vi "Sort Transposed Time Series Data.vi"(4 "Arrays in":dbl[][](array[numeric])) -> (1 "Arrays out":dbl[][](array[numeric]))   [LabVIEW 2013, in "Data Log Fetcher.lvlib"]
uses:
  Data Log Fetcher.lvlib
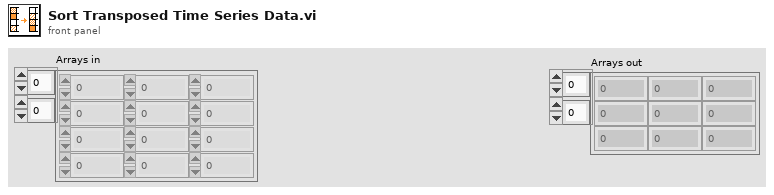
[diagram p1: front panel]
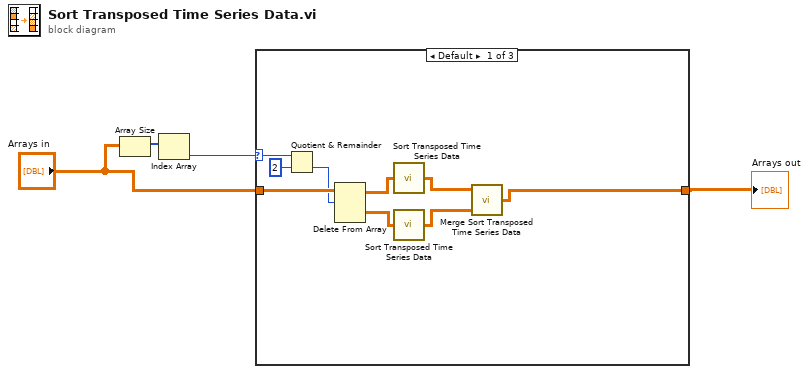
[diagram p0: block diagram]
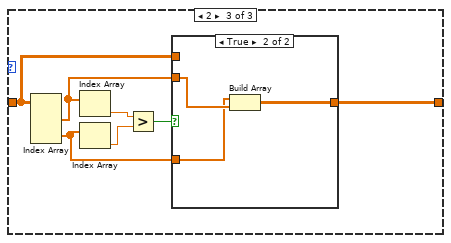
[diagram p3: hidden frame]
diagram:
  n1 = Array Size(array="Arrays in") -> (size(s)=w4:i32[])
  n2 = Index Array(array=w4) -> (element=w3:i32)  [unwired: 1 in]
  n3 = case shown="Default" w3 {
    selector: w3 -> [w12 _ _]
    tunnel: "Arrays in" -> [w13 w14 w15]
    tunnel: [w10 w14 w21] -> w2
    frame Default {
      n4 = Quotient & Remainder(x=w12, y=2) -> (floor(x/y)=w9:i32)  [unwired: 1 out]
      n5 = Delete From Array(array=w13, length=w9) -> (deleted portion=w7:dbl[][], array with subset deleted=w8:dbl[][])  [unwired: 2 in]
      n6 = call "Sort Transposed Time Series Data.vi"("Arrays in"=w8) -> ("Arrays out"=w6:dbl[][])  [unwired: 4 in]
      n7 = call "Sort Transposed Time Series Data.vi"("Arrays in"=w7) -> ("Arrays out"=w5:dbl[][])  [unwired: 4 in]
      n8 = call "Merge Sort Transposed Time Series Data.vi"("Time Series Array A"=w6, "Time Series Array B"=w5) -> ("Sorted Time Series Array"=w10:dbl[][])  [unwired: 5 in]
    }
    frame 1 {
    }
    frame 2 {
      n9 = Index Array(array=w15) -> (element #1=w17:dbl[], element #2=w16:dbl[])  [unwired: 4 in]
      n10 = Index Array(array=w17) -> (element=w19:dbl)  [unwired: 1 in]
      n11 = Index Array(array=w16) -> (element=w20:dbl)  [unwired: 1 in]
      n12 = Greater?(x=w19, y=w20) -> (0:w18:bool)
      n13 = case shown="True" w18 {
        tunnel: [w22 w25] -> w21
        tunnel: w17 -> [_ w24]
        tunnel: w16 -> [_ w23]
        tunnel: w15 -> [w22 _]
        frame False {
        }
        frame True {
          n14 = Build Array(w23, w24) -> (w25:dbl[][])
        }
      }
    }
  }
  "Arrays out" <- w2
